vi "Sel_match_from_StringArr.vi"(7 "Ignore case (TRUE def)":bool=TRUE, 10 "String to match":string="c:\\DATA", 11 "String Array In":string[](array[string])=["the settings file open properly", "Init", "the temperature file open properly", "astrocamInit: lodFile = C:\\vlt\\assembly\\h2rg-20141010\\SNAP\\tim_h2rg_SNAP.lod", "Getting device bindings ... done !", "Opening PCI driver ... ", "done!", "Calling astrocamConfig ", "astrocamConfig start ...", "Setting up controllerdone!", "Opening shutter ...", "Configuring ...", "RNT = 1", "OFA 0x1ec", "Waiting for image ..", "Done=true ", "GotImage - returning  ", "c:\\DATA\\20141011-102717-0.fits", "Got image.", "Waiting for image ..", "Done=true ", "GotImage - returning  ", "c:\\DATA\\20141011-102717-1.fits", "Got image.", "Close", "Test", "Done", ""]) -> (1 "Inx Exact match":i32[](array[numeric]), 2 "Inx matches":i32[](array[numeric]), 3 "String Array Matched":string[](array[string])=["c:\\DATA\\20141011-102717-0.fits", "c:\\DATA\\20141011-102717-1.fits"])   [LabVIEW 2011]
panel:
  out "Array Size":i32=2
  out "String Found Inx":i32[](array[numeric])=[-1, -1, -1, -1, -1, -1, -1, -1, -1, -1, -1, -1, -1, -1, -1, -1, -1, 0, -1, -1, -1, -1, 0, -1, -1, -1, -1, -1]
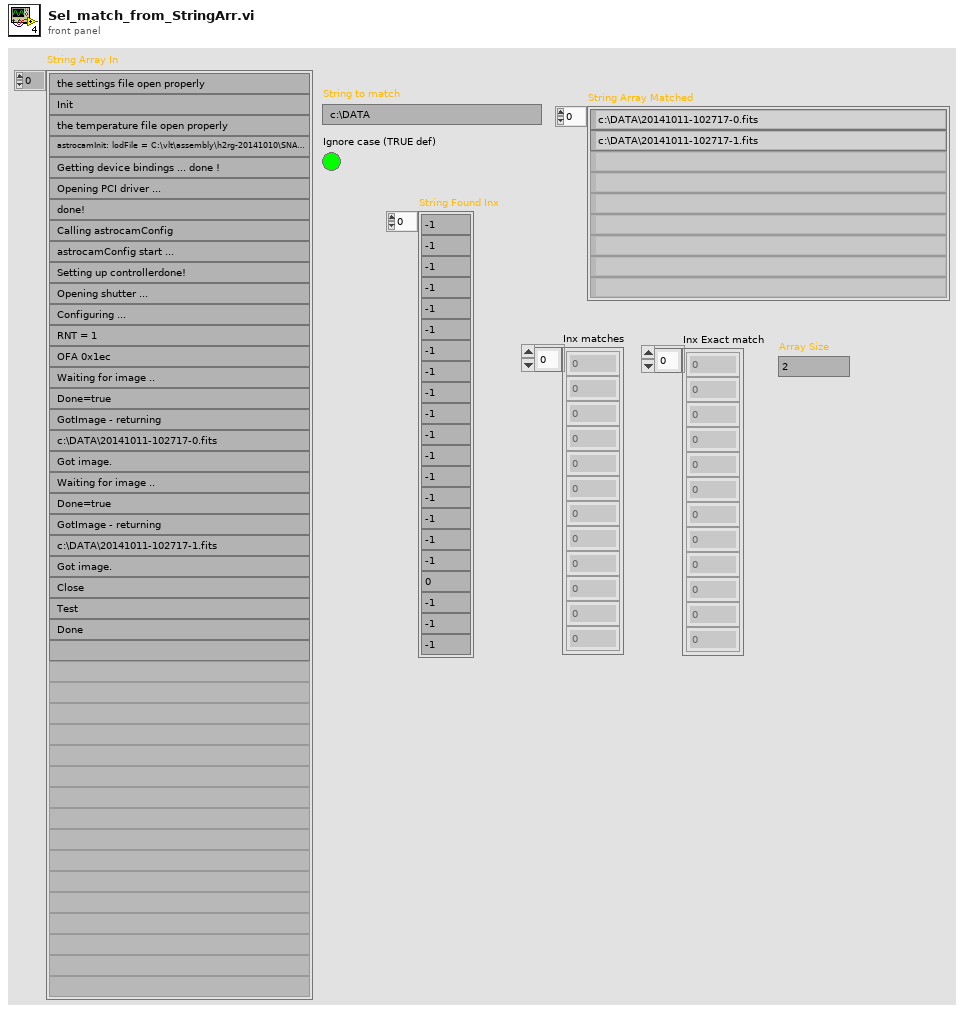
[diagram p1: front panel]
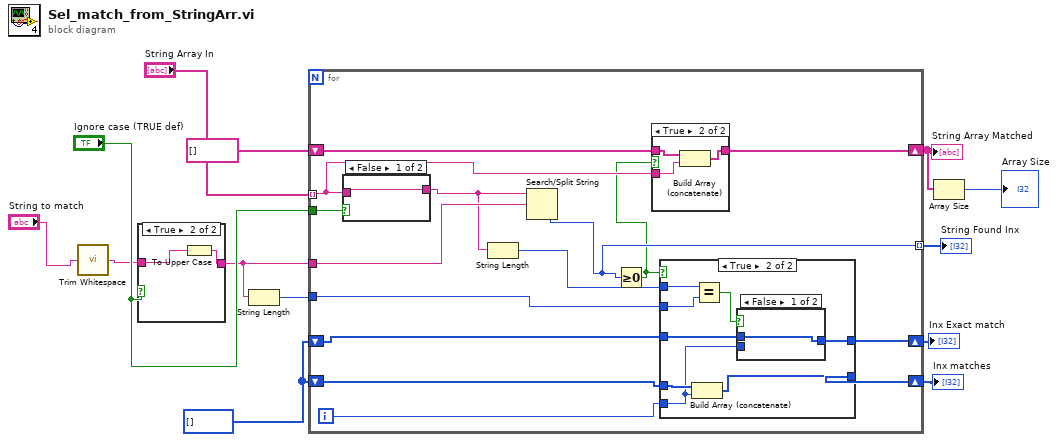
[diagram p0: block diagram]
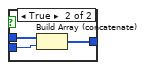
[diagram p4: hidden frame]
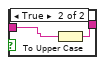
[diagram p5: hidden frame]
diagram:
  w2 = i32[] []
  n1 = call <vilib>:"Trim Whitespace.vi"("string"="String to match") -> ("trimmed string"=w6:string)  [unwired: 1 in]
  n2 = case shown="True" "Ignore case (TRUE def)" {
    tunnel: w6 -> [w14 w16]
    tunnel: [w14 w15] -> w5
    frame False {
    }
    frame True {
      n3 = To Upper Case(1:w16) -> (0:w15:string)
    }
  }
  n4 = String Length(string=w5) -> (length=w4:i32)
  n5 = for {
    tunnel: "String Array In" -> [w28] mode=indexing
    shift-right: [w31] -> w11
    shift-left: string[] [] -> [w30]
    tunnel: [w29] -> w12 mode=indexing
    tunnel: "Ignore case (TRUE def)" -> [w27]
    tunnel: w5 -> [w26]
    shift-right: [w19] -> w3
    shift-left: w2 -> [w23]
    tunnel: w4 -> [w22]
    shift-right: [w17] -> w1
    shift-left: w2 -> [w18]
    i -> [w24]
    n6 = case shown="False" w27 {
      tunnel: w28 -> [w46 w48]
      tunnel: [w46 w47] -> w21
      frame False {
      }
      frame True {
        n7 = To Upper Case(1:w48) -> (0:w47:string)
      }
    }
    n8 = String Length(string=w21) -> (length=w20:i32)
    n9 = Search/Split String(string=w21, search string/char (-)=w26) -> (offset of match=w29:i32)  [unwired: 1 in, 2 out]
    n10 = Greater Or Equal To 0?(x=w29) -> (x >= 0?=w25:bool)
    n11 = case shown="True" w25 {
      tunnel: w28 -> [_ w52]
      tunnel: [w49 w51] -> w31
      tunnel: w30 -> [w49 w50]
      frame False {
      }
      frame True {
        n12 = Build Array (concatenate)(w50, w52) -> (w51:string[])
      }
    }
    n13 = case shown="True" w25 {
      tunnel: [w33 w41] -> w19
      tunnel: w23 -> [w33 w40]
      tunnel: w24 -> [_ w34]
      tunnel: w22 -> [_ w38]
      tunnel: w20 -> [_ w39]
      tunnel: w18 -> [w32 w36]
      tunnel: [w32 w35] -> w17
      frame False {
      }
      frame True {
        n14 = Build Array (concatenate)(w40, w34) -> (w41:i32[])
        n15 = Equal?(x=w39, y=w38) -> (x = y?=w37:bool)
        n16 = case shown="False" w37 {
          tunnel: w36 -> [w42 w45]
          tunnel: [w42 w44] -> w35
          tunnel: w34 -> [_ w43]
          frame False {
          }
          frame True {
            n17 = Build Array (concatenate)(w45, w43) -> (w44:i32[])
          }
        }
      }
    }
  }
  "String Array Matched" <- w11
  "String Found Inx" <- w12
  "Inx matches" <- w3
  "Inx Exact match" <- w1
  n18 = Array Size(array=w11) -> (size(s)=→"Array Size":i32)
